vi "Get + Format Date + Time.vi"(8 "error in (no error)":errorcluster, 11 "Time":timestamp) -> (0 "error out":errorcluster, 2 "Time String [Local Time Format]":string, 3 "Date String [YYYY-MM-DD]":string)   [LabVIEW 2010]
panel:
  # "--- Outputs ---"
  # "--- Inputs ---"
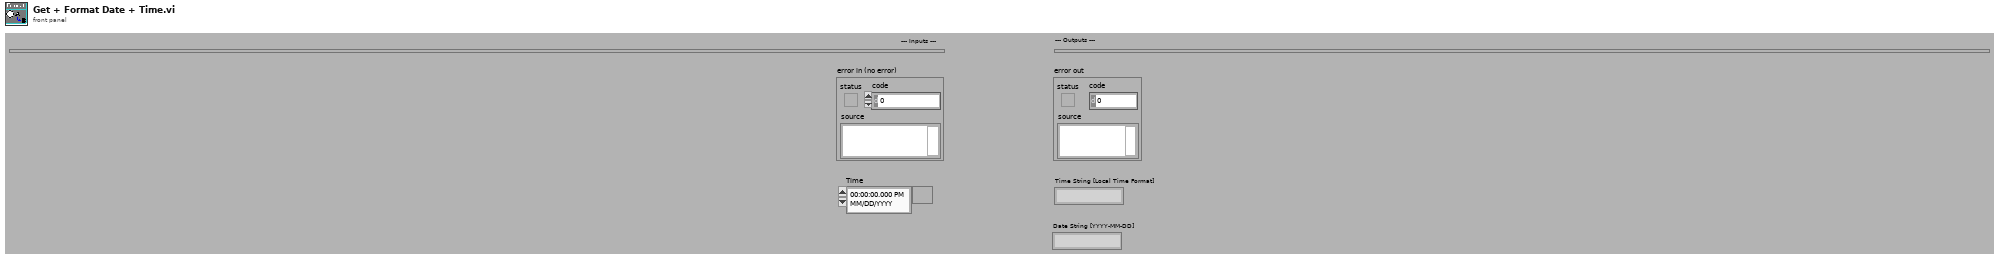
[diagram p1: front panel]
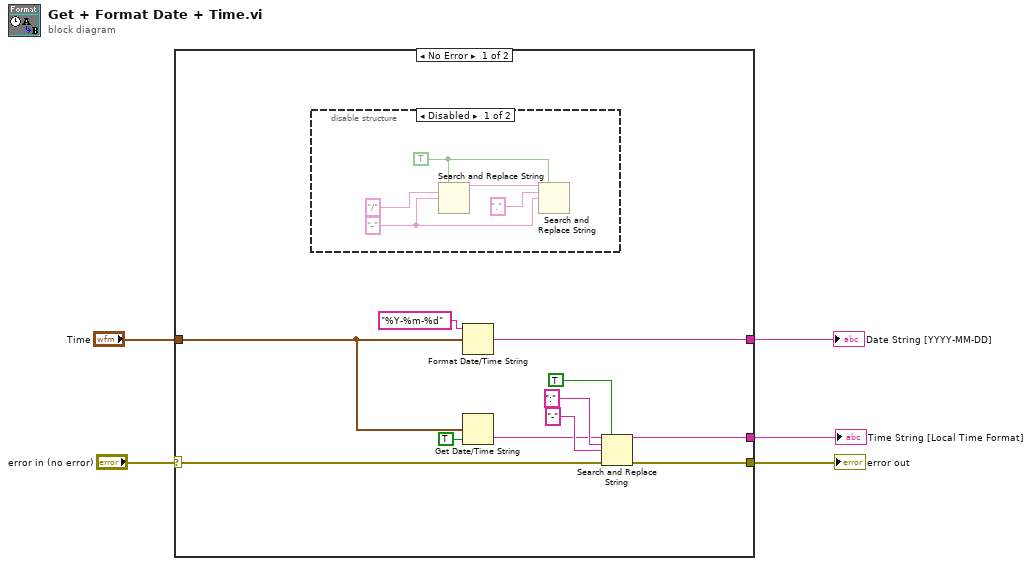
[diagram p0: block diagram]
diagram:
  n1 = case shown="No Error" "error in (no error)" {
    selector: "error in (no error)" -> [w10 w22]
    tunnel: [w9 w22] -> w4
    tunnel: [w8 _] -> w3
    tunnel: [w7 _] -> w2
    tunnel: "Time" -> [w6 _]
    frame No Error {
      n2 = disable-structure shown="Disabled" {
        frame Disabled {
          w17 = TRUE ("replace all? (F)")
          w20 = "-" ("replace string (\"\")")
          n3 = Search and Replace String(replace all?=w17, search string="/", replace string=w20) -> (result string=w19:string)  [unwired: 5 in, 3 out]
          n4 = Search and Replace String(replace all?=w17, input string=w19, search string=".", replace string=w20) -> ()  [unwired: 4 in, 4 out]
        }
        frame Enabled {
        }
      }
      n5 = Format Date/Time String(time format string (%c)="%Y-%m-%d", seconds (now)=w6) -> (date/time string=w8:string)  [unwired: 1 in]
      n6 = Get Date/Time String(seconds (now)=w6, want seconds? (F)=TRUE) -> (time string=w11:string)  [unwired: 1 in, 1 out]
      n7 = Search and Replace String(replace all?=TRUE ("replace all? (F)"), input string=w11, search string=":", replace string="-" ("replace string (\"\")"), error in=w10) -> (result string=w7:string, error out=w9:errorcluster)  [unwired: 3 in, 2 out]
    }
    frame Error {
    }
  }
  "error out" <- w4
  "Time String [Local Time Format]" <- w2
  "Date String [YYYY-MM-DD]" <- w3
